vi "Driver - DTACQ - Initialise TCP Connection.vi"(7 "Description":string, 8 "Termination Character":string, 9 "timeout (ms)":i32, 10 "Port":u16, 11 "Address":string) -> (3 "DTACQ Connection Data Out":T1={"Description"="", "Address"="", "Port"=0, "timeout (ms)"=5000, "Termination Character"="\n", "TCP Connection Reference"=refnum, "Open Connection"=FALSE})   [LabVIEW 2017, in "Communications Library.lvlib"]
doc: "Initialises a TCP connection to a DTACQ device.\n\nSets the value of the DTACQ Connection Data Cluster. \nAfter initialising the connect, in must be opened in order to send data."
uses:
  Communications Library.lvlib
  Typedefs/DTACQ Connection Data--Cluster.ctl
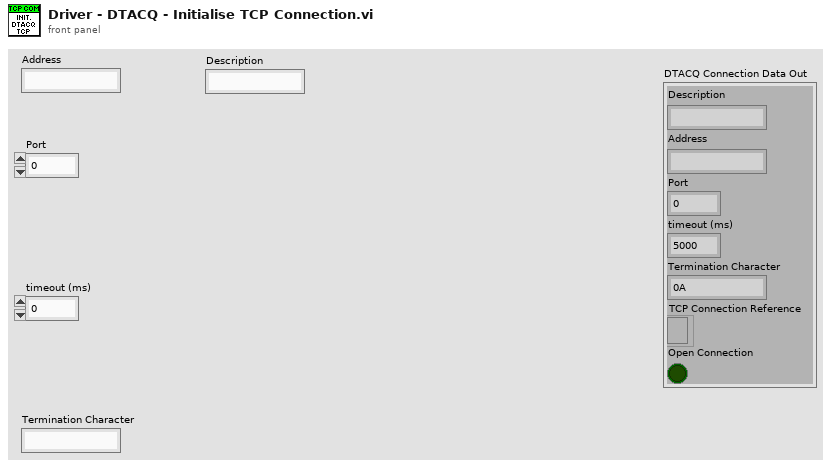
[diagram p1: front panel]
types:
  T1 = typedef "Communications Library.lvlib/DTACQ Connection Data--Cluster.ctl" = cluster{"Description":string, "Address":string, "Port":u16, "timeout (ms)":i32, "Termination Character":string, "TCP Connection Reference":refnum<k5>, "Open Connection":bool}
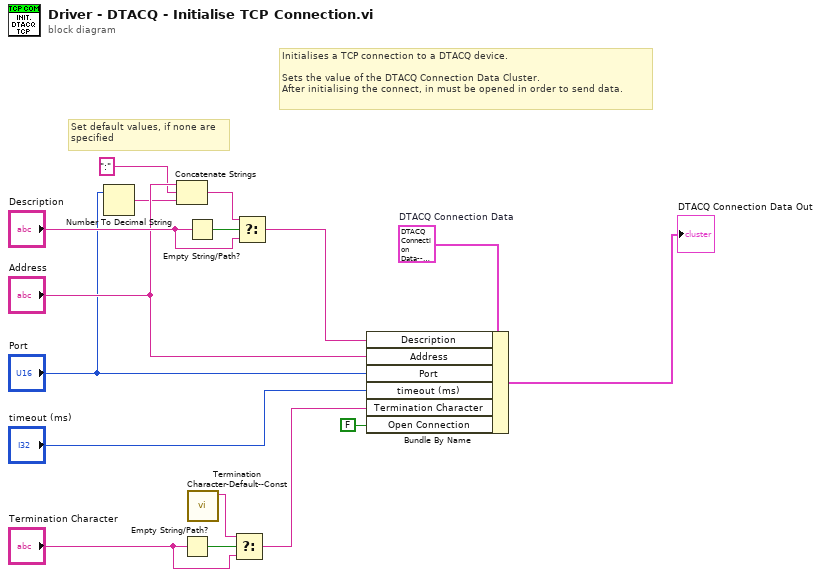
[diagram p0: block diagram]
diagram:
  w16 = T1 {"Description"="", "Address"="", "Port"=0, "timeout (ms)"=5000, "Termination Character"="\n", "TCP Connection Reference"=refnum, "Open Connection"=FALSE}  # DTACQ Connection Data
  # "Initialises a TCP connection to a DTACQ device.\n\nSets the value of the DTACQ Connection Data Cluster.  \nAfter initialising the connect, in must be opened in order to send data."
  # "Set default values, if none are \nspecified"
  n1 = Number To Decimal String(number="Port") -> (decimal integer string=w4:string)  [unwired: 1 in]
  n2 = Concatenate Strings("Address", ":" ("string"), w4) -> (w2:string)
  n3 = Empty String/Path?(string/path="Termination Character") -> (empty?=w13:bool)
  n4 = Empty String/Path?(string/path="Description") -> (empty?=w8:bool)
  n5 = call "Termination Character-Default--Const.vi"() -> ("Termination Character"=w12:string)  [unwired: 11 in]
  n6 = Select(t=w12, s=w13, f="Termination Character") -> (s? t:f=w10:string)
  n7 = Select(t=w2, s=w8, f="Description") -> (s? t:f=w7:string)
  n8 = Bundle By Name(cluster=w16, "Description"=w7, "Address"="Address", "Port"="Port", "timeout (ms)"="timeout (ms)", "Termination Character"=w10, "Open Connection"=FALSE) -> (→"DTACQ Connection Data Out":T1)
